vi "Enqueue-Command-SetDataMember.vi"(6 "Timeout [ms] (-1)":i32=-1, 7 "Has Priority (F)":bool, 8 "error in (no error)":errorcluster, 9 "Data Member Value":variant, 10 "Data Member":T1, 11 "Engine in":refnum<class "Engine.lvclass">) -> (0 "error out":errorcluster, 2 "Timeout?":bool, 3 "Engine out":refnum<class "Engine.lvclass">)   [LabVIEW 2024, in "GLF.lvlib" / "Engine.lvclass"]
uses:
  Engine.lvclass
  Engine.lvclass/Engine.ctl
  Command--enum.ctl
  DataMember--enum.ctl
  CommandData-SetDataMember--cluster.ctl
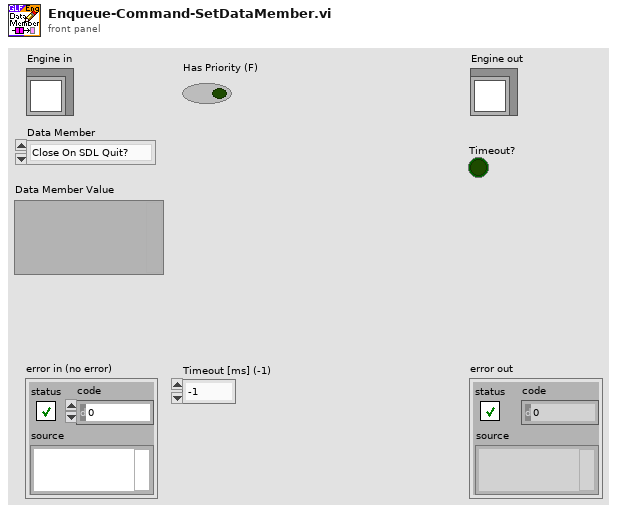
[diagram p1: front panel]
types:
  T1 = typedef "GLF.lvlib/Engine.lvclass/DataMember--enum.ctl" = enum16{"Close On SDL Quit?"}
  T2 = typedef "GLF.lvlib/Engine.lvclass/CommandData-SetDataMember--cluster.ctl" = cluster{"Data Member":T1, "Value":variant}
  T3 = typedef "GLF.lvlib/Engine.lvclass/Command--enum.ctl" = enum16{"Quit", "Set Data Member"}
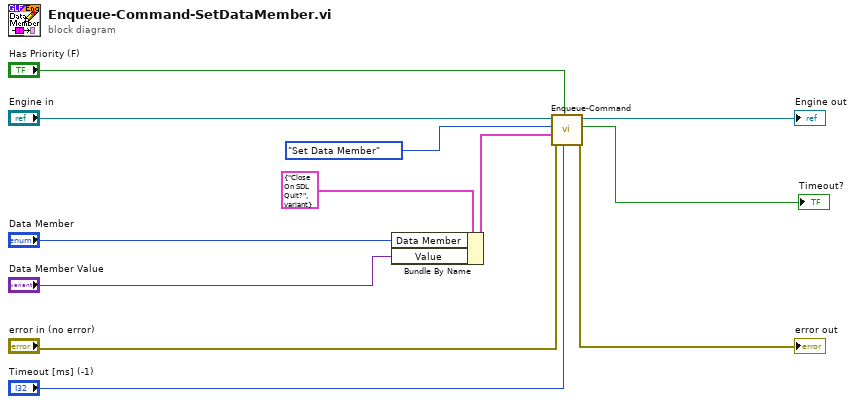
[diagram p0: block diagram]
diagram:
  n1 = Bundle By Name(cluster=T2 {"Data Member"=enum."Close On SDL Quit?", "Value"=variant} ("Set Data Member Cmd Data"), "Data Member"="Data Member", "Value"="Data Member Value") -> (w4:T2)
  n2 = call "Enqueue-Command.vi"("Timeout [ms] (-1)"="Timeout [ms] (-1)", "Has Priority (F)"="Has Priority (F)", "error in (no error)"="error in (no error)", "Cmd Data"=w4, "Cmd"=Command--enum."Set Data Member", "Engine in"="Engine in") -> ("error out"=→"error out":errorcluster, "Timeout?"=→"Timeout?":bool, "Engine out"=→"Engine out":refnum<class "Engine.lvclass">)  [unwired: 3 in]
